vi "ExtractFlagBits.vi"(11 "Fixed Header":u8 format="%08b") -> (0 "Valid QoS":bool, 1 "RETAIN":bool, 2 "QoS":T1, 3 "DUP":bool)   [LabVIEW 2013, in "PUBLISH.lvclass"]
uses:
  PUBLISH.lvclass
  ControlPacket/QualityOfService -- enum.ctl
  ControlPacket/ControlPacket.lvclass
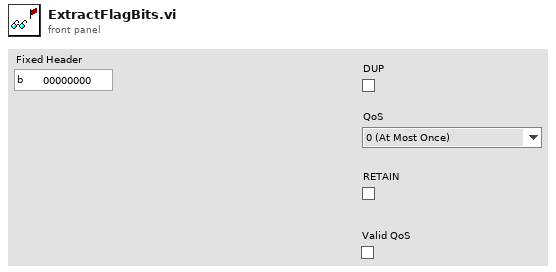
[diagram p1: front panel]
types:
  T1 = typedef "ControlPacket.lvclass/QualityOfService -- enum.ctl" = enum16{"0 (At Most Once)", "1 (At Least Once)", "2 (Exactly Once)"}
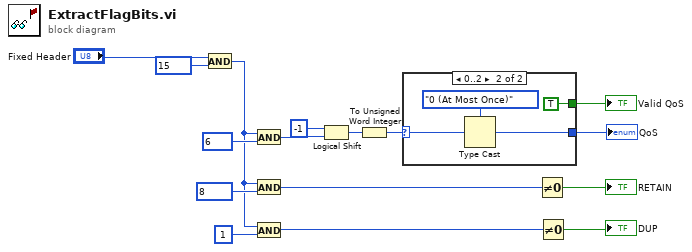
[diagram p0: block diagram]
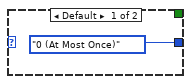
[diagram p2: hidden frame]
diagram:
  n1 = And(x="Fixed Header", y=u8 15) -> (x .and. y?=w3:u8)
  n2 = And(x=w3, y=u8 6) -> (x .and. y?=w11:u8)
  n3 = And(x=w3, y=u8 8) -> (x .and. y?=w5:u8)
  n4 = And(x=w3, y=u8 1) -> (x .and. y?=w4:u8)
  n5 = Logical Shift(y=i16 -1, x=w11) -> (x << y=w10:u8)
  n6 = To Unsigned Word Integer(number=w10) -> (unsigned 16bit integer=w2:u16)
  n7 = case shown="0..2" w2 {
    selector: w2 -> [_ w19]
    tunnel: [QualityOfService_--_enum."0 (At Most Once)" ("QoS") w21] -> w13
    tunnel: [_ TRUE] -> w1
    frame Default {
    }
    frame 0..2 {
      n8 = Type Cast(type=QualityOfService_--_enum."0 (At Most Once)" ("QoS"), x=w19) -> (*(type *) &x=w21:T1)
    }
  }
  "QoS" <- w13
  "Valid QoS" <- w1
  n9 = Not Equal To 0?(x=w5) -> (x != 0?=→"RETAIN":bool)
  n10 = Not Equal To 0?(x=w4) -> (x != 0?=→"DUP":bool)
